vi "Start Running.vi"(8 "error in (no error)":errorcluster, 11 "CIFCorePlugin in":refnum<class "CIFCorePlugin.lvclass">) -> (0 "error out":errorcluster, 3 "CIFCorePlugin out":refnum<class "CIFCorePlugin.lvclass">)   [LabVIEW 2021, in "CIFCorePlugin.lvclass"]
doc: "Update the timestamp. Time is U64, absolute time in nS in the appropriate clockID configured for the plugin. If a 0 is wired it will automatically get the current time."
uses:
  CIFCorePlugin.lvclass
  CIFCorePlugin.lvclass/CIFCorePlugin.ctl
  <vilib>/CIF Foundation/CIF Utilities/Time/Typedef/Future Time Event Limits.ctl
  <vilib>/CIF Foundation/CIF Utilities/Time/SubVIs/Add Error.vi
  <vilib>/CIF Foundation/CIF Utilities/Time/System Time/LabVIEW Time to TAI Time.vi
  <vilib>/CIF Foundation/CIF Utilities/Errors/Append Error Location.vi
  <vilib>/CIF Foundation/CIF Utilities/Time/Time_CIF_U.lvlib
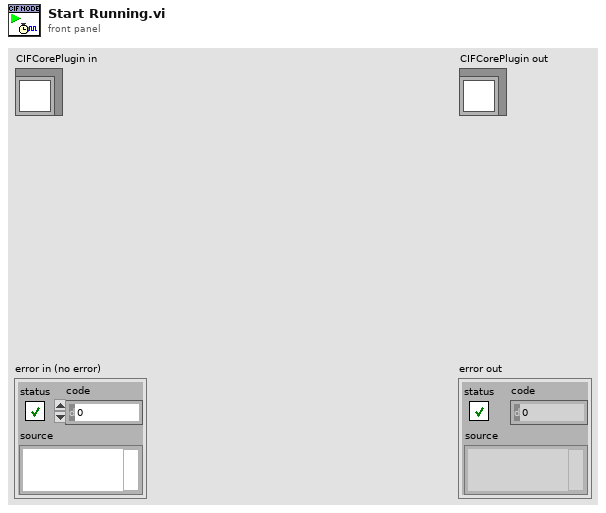
[diagram p1: front panel]
types:
  T1 = typedef "Time_CIF_U.lvlib/Future Time Event Limits.ctl" = cluster{"Maximum":i64, "Minimum":i64}
  T2 = typedef "CIFCorePlugin.lvclass/Energized States.ctl" = enum16{"Listen", "Prepare", "Execute", "Housekeep", "Cleanup", "Destroy"}
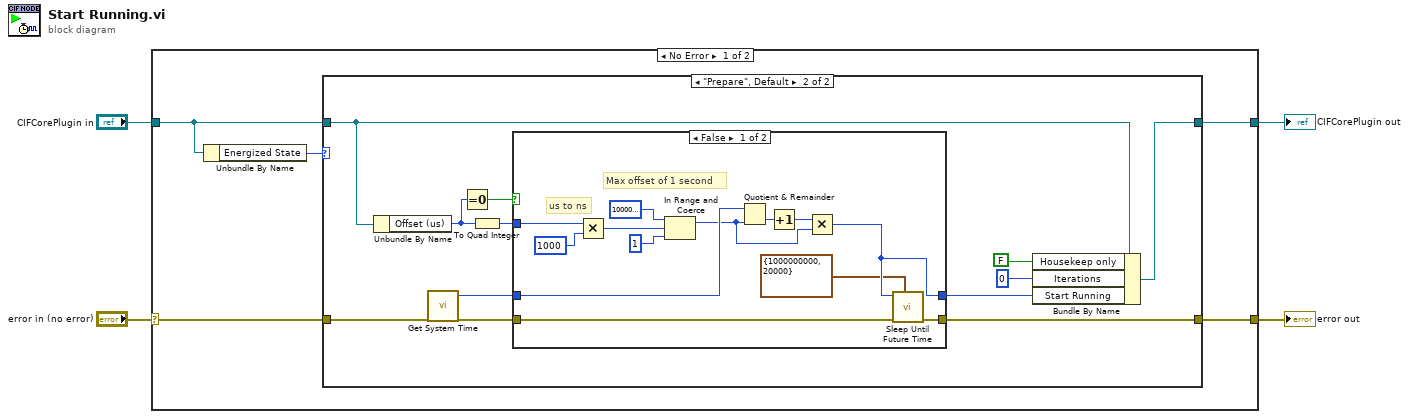
[diagram p0: block diagram]
diagram:
  n1 = case shown="No Error" "error in (no error)" {
    selector: "error in (no error)" -> [w7 w38]
    tunnel: [w8 w38] -> w3
    tunnel: [w9 w39] -> w1
    tunnel: "CIFCorePlugin in" -> [w6 w39]
    frame No Error {
      n2 = Unbundle By Name(w6) -> ("Energized State"=w5:T2)
      n3 = case shown="\"Prepare\", Default" w5 {
        tunnel: [w11 w22] -> w9
        tunnel: [w10 w17] -> w8
        tunnel: w7 -> [w10 w12]
        tunnel: w6 -> [w11 w14]
        frame "Destroy" {
        }
        frame "Prepare", Default {
          n4 = Unbundle By Name(w14) -> ("Offset (us)"=w19:i32)
          n5 = call <vilib>:"Get System Time.vi"() -> ("Time (ns)"=w13:i64)  [unwired: 5 in]
          n6 = Equal To 0?(x=w19) -> (x = 0?=w20:bool)
          n7 = To Quad Integer(1:w19) -> (0:w18:i64)
          n8 = case shown="False" w20 {
            tunnel: w13 -> [w33 w37]
            tunnel: [w24 w37] -> w21
            tunnel: w18 -> [w32 _]
            tunnel: w12 -> [w26 w36]
            tunnel: [w25 w36] -> w17
            frame False {
              # "us to ns"
              # "Max offset of 1 second"
              n9 = Multiply(x=w32, y=i64 1000) -> (x*y=w30:i64)
              n10 = In Range and Coerce(upper limit=i64 1000000000, x=w30, lower limit=i64 1) -> (coerced(x)=w27:i64)  [unwired: 1 out]
              n11 = Quotient & Remainder(x=w33, y=w27) -> (floor(x/y)=w29:i64)  [unwired: 1 out]
              n12 = Increment(x=w29) -> (x+1=w28:i64)
              n13 = Multiply(x=w28, y=w27) -> (x*y=w24:i64)
              n14 = call <vilib>:"Sleep Until Future Time.vi"("FTE Limits (ns)"=T1 {"Maximum"=1000000000, "Minimum"=20000}, "error in (no error)"=w26, "Wake Time (ns)"=w24) -> ("error out"=w25:errorcluster)  [unwired: 6 in, 2 out]
            }
            frame True {
            }
          }
          n15 = Bundle By Name(cluster=w14, "Housekeep only"=FALSE ("Running Internal Data.Housekeep only"), "Iterations"=i64 0, "Start Running"=w21) -> (w22:refnum<class "CIFCorePlugin.lvclass">)
        }
      }
    }
    frame Error {
    }
  }
  "error out" <- w3
  "CIFCorePlugin out" <- w1
